vi "GUI.vi"(9 "GUI Builder in":refnum<class "GUI Builder.lvclass">) -> ()   [LabVIEW 2021, in "App-Builder Library.lvlib" / "GUI Builder.lvclass"]
uses:
  GUI Builder.lvclass
  GUI Builder.lvclass/GUI Builder.ctl
  Builder/Builder.lvclass
  Builder/Build Type.ctl
  Builder/App descriptions.ctl
panel:
  in  "Application found":T1[](array[typedef])
  out "update":bool
  in  "Build button":bool
  # "Build Name"
  # "Type"
  # "Current Version"
  # "Next Version"
  # "Build?"
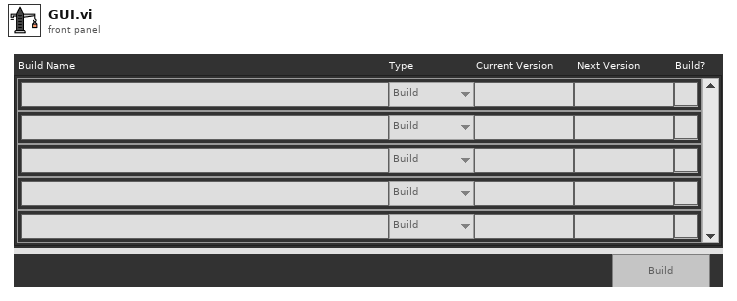
[diagram p1: front panel]
types:
  T1 = typedef "App-Builder Library.lvlib/Builder.lvclass/App descriptions.ctl" = cluster{"App Name":string, "Build Type":T2, "Current Version":string, "Next Version":string, "Check":bool}
  T2 = typedef "App-Builder Library.lvlib/Builder.lvclass/Build Type.ctl" = enum16{"Major", "Minor", "Fix", "Build"}
  T3 = enum8{"Enabled", "Disabled", "Disabled and Grayed Out"}
  T4 = typedef "NI_App_Builder_API.lvlib/Build Specification Version.ctl" = cluster{"Major":u16, "Minor":u16, "Fix":u16, "Build":u16}
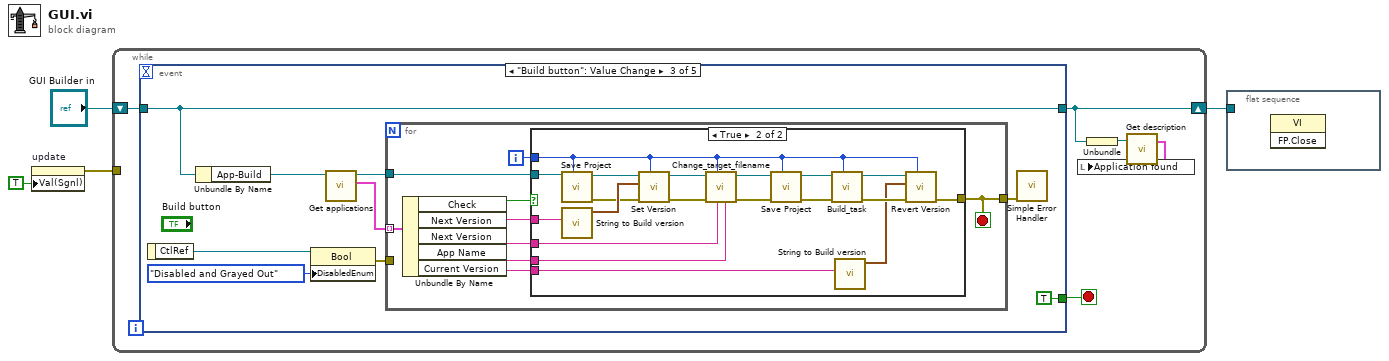
[diagram p0: block diagram]
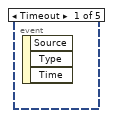
[diagram p2: hidden frame]
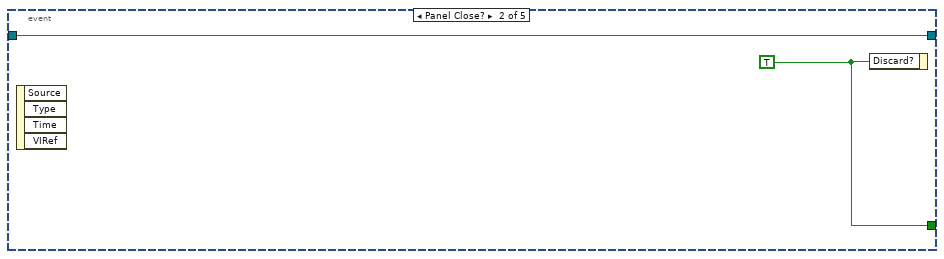
[diagram p3: hidden frame]
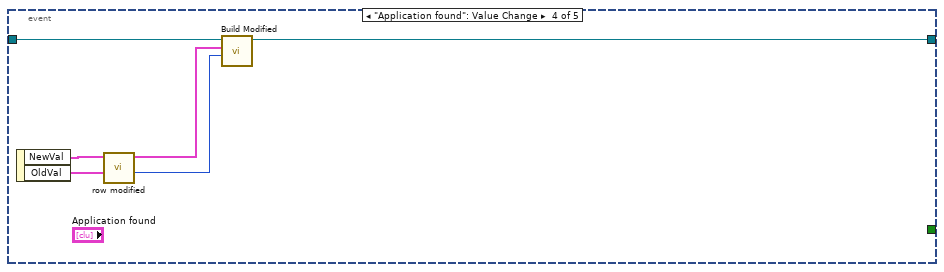
[diagram p5: hidden frame]
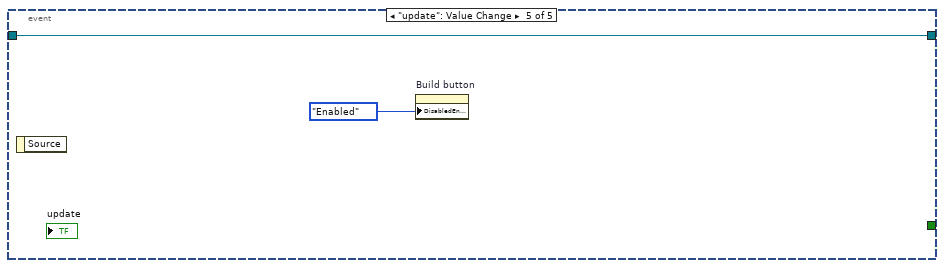
[diagram p6: hidden frame]
diagram:
  n1 = property on="update" class="Bool (strict)"("Val(Sgnl)"=TRUE ("Value (Signaling)")) -> (error out=w2:errorcluster)  [unwired: 2 in, 1 out]
  n2 = while {
    shift-right: [w6] -> w1
    shift-left: "GUI Builder in" -> [w8]
    tunnel: w2 -> [_]
    stop <- w9 stop-if-true
    n3 = event shown="[2] \"Build button\": Value Change" {
      selector: _ -> [_ _ _ _ _]
      dyn-events: _ -> [_ _ _ _ _]
      timeout: _ -> [_ _ _ _ _]
      tunnel: [_ w11 TRUE ("Discard?") _ _] -> w9
      tunnel: w8 -> [_ w10 w20 w52 w56]
      tunnel: [_ w10 w20 w50 w56] -> w6
      event Timeout {
        n4 = event-data() -> ()  [unwired: 1 in, 3 out]
      }
      event Panel Close? {
        w11 = TRUE ("Discard?")
        n5 = event-data() -> ()  [unwired: 1 in, 4 out]
        n6 = event-data("Discard?"=w11) -> ()  [unwired: 1 in, 1 out]
      }
      event "Build button": Value Change {
        n7 = event-data() -> ("CtlRef"=w16:refnum<vi>)  [unwired: 1 in]
        n8 = Unbundle By Name(w20) -> ("App-Build"=w19:refnum<class "Builder.lvclass">)
        n9 = property class="Bool"(reference=w16, "DisabledEnum"=T3."Disabled and Grayed Out" ("Disabled")) -> (error out=w14:errorcluster)  [unwired: 1 in, 1 out]
        n10 = call "Get applications.vi"("Builder in"=w19) -> ("Applications"=w17:T1[], "Builder out"=w18:refnum<class "Builder.lvclass">)  [unwired: 9 in]
        n11 = for {
          tunnel: [w24] -> w12
          tunnel: w18 -> [w29]
          tunnel: w17 -> [w28] mode=indexing
          tunnel: w14 -> [_]
          i -> [w26]
          stop <- w24 stop-if-true
          n12 = Unbundle By Name(w28) -> ("Check"=w27:bool, "Next Version"=w25:string, "Next Version"=w22:string, "App Name"=w23:string, "Current Version"=w21:string)
          n13 = case shown="True" w27 {
            tunnel: [_ w32] -> w24
            tunnel: w29 -> [_ w44]
            tunnel: w26 -> [_ w34]
            tunnel: w25 -> [_ w46]
            tunnel: w23 -> [_ w37]
            tunnel: w22 -> [_ w36]
            tunnel: w21 -> [_ w31]
            frame False {
            }
            frame True {
              n14 = call "Save Project.vi"("index"=w34, "Builder in"=w44) -> ("error out"=w38:errorcluster, "Builder out"=w43:refnum<class "Builder.lvclass">)  [unwired: 8 in]
              n15 = call "String to Build version.vi"("Build Version (String)"=w46) -> ("Build Version"=w45:T4)  [unwired: 10 in]
              n16 = call "Set Version.vi"("Index"=w34, "error in"=w38, "Build Version"=w45, "Builder in"=w43) -> ("error out"=w47:errorcluster, "Builder out"=w48:refnum<class "Builder.lvclass">)  [unwired: 6 in]
              n17 = call "Change_target_filename.vi"("App Name"=w37, "New Version"=w36, "index"=w34, "error in (no error)"=w47, "Builder in"=w48) -> ("error out"=w42:errorcluster, "Builder out"=w41:refnum<class "Builder.lvclass">)  [unwired: 5 in]
              n18 = call "Save Project.vi"("index"=w34, "error in"=w42, "Builder in"=w41) -> ("error out"=w39:errorcluster, "Builder out"=w40:refnum<class "Builder.lvclass">)  [unwired: 7 in]
              n19 = call "Build_task.vi"("index"=w34, "error in"=w39, "Builder in"=w40) -> ("error out"=w33:errorcluster, "Builder out"=w35:refnum<class "Builder.lvclass">)  [unwired: 6 in, 1 out]
              n20 = call "String to Build version.vi"("Build Version (String)"=w31) -> ("Build Version"=w30:T4)  [unwired: 10 in]
              n21 = call "Revert Version.vi"("Index"=w34, "error in"=w33, "Build Version"=w30, "Builder in"=w35) -> ("error out"=w32:errorcluster)  [unwired: 6 in, 1 out]
            }
          }
        }
        n22 = call <vilib>:"Simple Error Handler.vi"("error in (no error)"=w12) -> ()  [unwired: 4 in, 5 out]
      }
      event "Application found": Value Change {
        n23 = event-data() -> ("NewVal"=w54:T1[], "OldVal"=w53:T1[])  [unwired: 1 in]
        n24 = call "row modified.vi"("OldVal"=w53, "NewVal"=w54) -> ("Index"=w49:i32, "Value Modified"=w51:T1)  [unwired: 8 in]
        n25 = call "Build Modified.vi"("index"=w49, "build modified"=w51, "GUI Builder in"=w52) -> ("GUI Builder out"=w50:refnum<class "GUI Builder.lvclass">)  [unwired: 8 in]
      }
      event "update": Value Change {
        n26 = event-data() -> ()  [unwired: 1 in, 1 out]
        n27 = property on="Build button" class="Bool"("DisabledEnum"=T3."Enabled" ("Disabled")) -> ()  [unwired: 2 in, 2 out]
      }
    }
    n28 = Unbundle(w6) -> (w5:refnum<class "Builder.lvclass">)
    n29 = call "Get description.vi"("Builder in"=w5) -> ("Applications"=w7:T1[])  [unwired: 2 in]
    n30 = local write "Application found"(w7) -> ()
  }
  n31 = flat-sequence {
    tunnel: w1 -> [_]
    frame #0 {
      n32 = invoke class="VI" method="FP.Close"() -> ()  [unwired: 3 in, 3 out]
    }
  }
